vi "rvc Euler to Rotation Matrix.vi"(6 "type of transformation":u16(ring) items=["active (alibi)", "passive (alias)"], 9 "type of rotations":u16(ring) items=["Extrinsic", "Intrinsic"], 10 "rotation order":T1=11 items=["X-Y-Z", "X-Z-Y", "Y-X-Z", "Y-Z-X", "Z-X-Y", "Z-Y-X", "X-Y-X", "X-Z-X", "Y-X-Y", "Y-Z-Y", "Z-X-Z", "Z-Y-Z"], 11 "euler angles":cluster{"phi":dbl, "theta":dbl, "psi":dbl}) -> (0 "error":i32, 3 "rotation matrix":T2)   [LabVIEW 2013]
uses:
  <vilib>/Analysis/Matrix/Datatypes/RealMatrix.ctl
  <vilib>/Analysis/coordinate.llb/Euler Rotation Order.ctl
  <vilib>/Analysis/NI_AALPro.lvlib
  <vilib>/Analysis/Matrix/NI_Matrix.lvlib
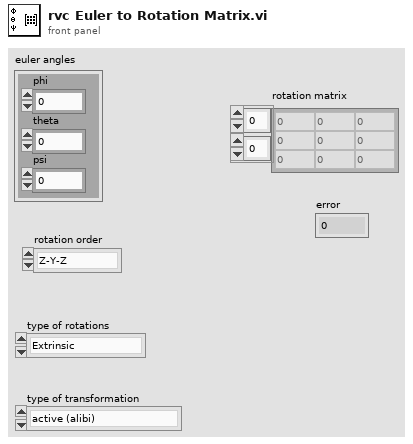
[diagram p1: front panel]
types:
  T1 = typedef "NI_AALPro.lvlib/Euler Rotation Order.ctl" = u16
  T2 = typedef "NI_Matrix.lvlib/RealMatrix.ctl" = dbl[][]
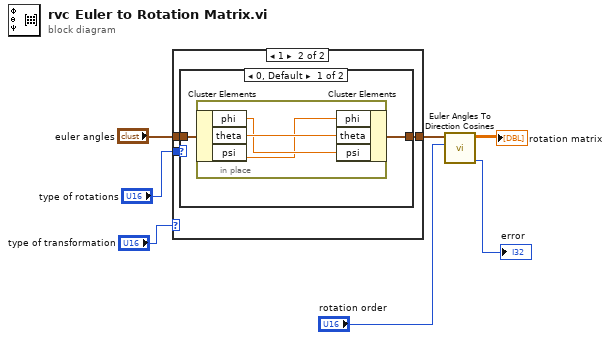
[diagram p0: block diagram]
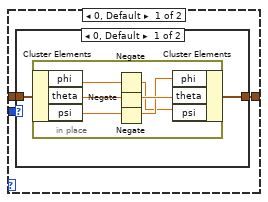
[diagram p2: hidden frame]
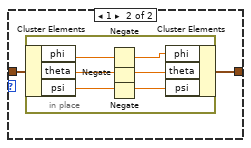
[diagram p3: hidden frame]
diagram:
  n1 = case shown="1" "type of transformation" {
    tunnel: [w10 w29] -> w7
    tunnel: "euler angles" -> [w9 w28]
    tunnel: "type of rotations" -> [w8 w27]
    frame 0, Default {
      n2 = case shown="0, Default" w8 {
        tunnel: [w12 w20] -> w10
        tunnel: w9 -> [w11 w19]
        frame 0, Default {
          n3 = in-place {
            n4 = in-place-cluster #1(w11) -> ("phi"=w17:dbl, "theta"=w18:dbl, "psi"=w16:dbl)
            n5 = Negate(x=w17) -> (-x=w13:dbl)
            n6 = Negate(x=w18) -> (-x=w15:dbl)
            n7 = Negate(x=w16) -> (-x=w14:dbl)
            n8 = in-place-cluster #1("phi"=w14, "theta"=w15, "psi"=w13) -> (w12:cluster{"phi":dbl, "theta":dbl, "psi":dbl})
          }
        }
        frame 1 {
          n9 = in-place {
            n10 = in-place-cluster #2(w19) -> ("phi"=w25:dbl, "theta"=w26:dbl, "psi"=w24:dbl)
            n11 = Negate(x=w25) -> (-x=w21:dbl)
            n12 = Negate(x=w26) -> (-x=w23:dbl)
            n13 = Negate(x=w24) -> (-x=w22:dbl)
            n14 = in-place-cluster #2("phi"=w21, "theta"=w23, "psi"=w22) -> (w20:cluster{"phi":dbl, "theta":dbl, "psi":dbl})
          }
        }
      }
    }
    frame 1 {
      n15 = case shown="0, Default" w27 {
        tunnel: [w31 w35] -> w29
        tunnel: w28 -> [w30 w35]
        frame 0, Default {
          n16 = in-place {
            n17 = in-place-cluster #3(w30) -> ("phi"=w33:dbl, "theta"=w34:dbl, "psi"=w32:dbl)
            n18 = in-place-cluster #3("phi"=w32, "theta"=w34, "psi"=w33) -> (w31:cluster{"phi":dbl, "theta":dbl, "psi":dbl})
          }
        }
        frame 1 {
        }
      }
    }
  }
  n19 = call <vilib>:"Euler Angles To Direction Cosines.vi"("rotation order"="rotation order", "Euler Angles"=w7) -> ("error"=→"error":i32, "Direction Cosines"=→"rotation matrix":dbl[][])  [unwired: 8 in]
